vi "Transfer Multiple.vi"() -> ()   [LabVIEW 2020, in "Examples.lvlib"]
uses:
  Examples.lvlib
  Network Config/Network Config.lvclass
  Server Config/Server Config.lvclass
  PropertyBinder/Binding/Binding.lvclass/Binding.ctl
  PropertyBinder/Binding/Transfer.vi
  PropertyBinder/Binding/Set.vi
  PropertyBinder/Binding/Get.vi
  PropertyBinder/Binding/Binding.lvclass
panel:
  out "Time":dbl
  out "error out":errorcluster
  out "Bind Port":u16
  out "Bind Address":string
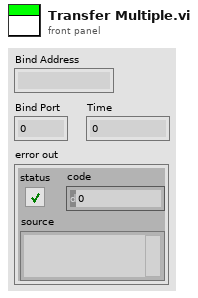
[diagram p1: front panel]
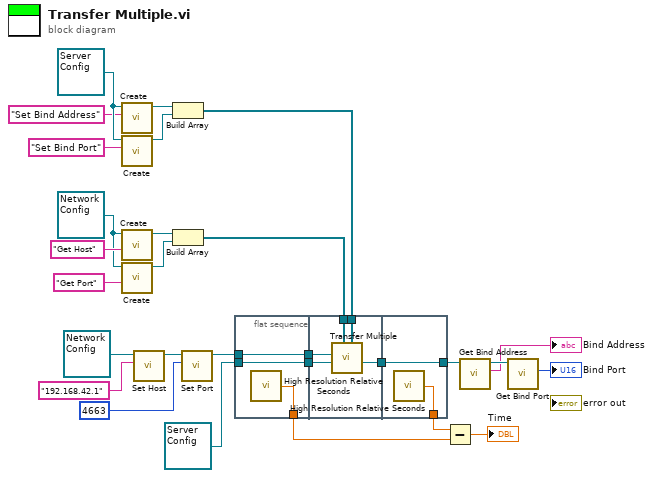
[diagram p0: block diagram]
diagram:
  w25 = refnum<class "Server Config.lvclass"> refnum ("Examples.lvlib:Server Config.lvclass")
  w26 = refnum<class "Network Config.lvclass"> refnum ("Examples.lvlib:Network Config.lvclass")
  n1 = call "Create.vi"("Setter VI Name"="Set Bind Address" ("Getter VI Name"), "Class Type"=w25) -> ("Binding out"=w11:refnum<class "Binding.lvclass">)  [unwired: 8 in, 1 out]
  n2 = call "Create.vi"("Setter VI Name"="Set Bind Port", "Class Type"=w25) -> ("Binding out"=w10:refnum<class "Binding.lvclass">)  [unwired: 8 in, 1 out]
  n3 = call "Create.vi"("Getter VI Name"="Get Host", "Class Type"=w26) -> ("Binding out"=w13:refnum<class "Binding.lvclass">)  [unwired: 8 in, 1 out]
  n4 = call "Create.vi"("Getter VI Name"="Get Port", "Class Type"=w26) -> ("Binding out"=w12:refnum<class "Binding.lvclass">)  [unwired: 8 in, 1 out]
  n5 = call "Set Host.vi"("Host"="192.168.42.1", "Network Config in"=refnum<class "Network Config.lvclass"> refnum ("Examples.lvlib:Network Config.lvclass")) -> ("Network Config out"=w20:refnum<class "Network Config.lvclass">)  [unwired: 8 in, 1 out]
  n6 = Build Array(w11, w10) -> (w8:refnum<class "Binding.lvclass">[])
  n7 = Build Array(w13, w12) -> (w9:refnum<class "Binding.lvclass">[])
  n8 = call "Set Port.vi"("Port"=u16 4663, "Network Config in"=w20) -> ("Network Config out"=w15:refnum<class "Network Config.lvclass">)  [unwired: 8 in, 1 out]
  n9 = flat-sequence {
    tunnel: refnum<class "Server Config.lvclass"> refnum ("Examples.lvlib:Server Config.lvclass") -> [w30]
    tunnel: w15 -> [w31]
    tunnel: [w31] -> w6
    tunnel: [w30] -> w5
    tunnel: [w29] -> w2
    tunnel: w9 -> [w34]
    tunnel: w8 -> [w33]
    tunnel: w6 -> [w36]
    tunnel: w5 -> [w35]
    tunnel: [w32] -> w4
    tunnel: [w38] -> w7
    tunnel: w4 -> [w38]
    tunnel: [w37] -> w3
    frame #0 {
      n10 = call <vilib>:"High Resolution Relative Seconds.vi"() -> ("relative seconds"=w29:dbl)
    }
    frame #1 {
      n11 = call "Transfer Multiple.vi"("To Bindings"=w33, "From Bindings"=w34, "To Class in"=w35, "From Class in"=w36) -> ("To Class out"=w32:refnum<class "Server Config.lvclass">)  [unwired: 5 in, 2 out]
    }
    frame #2 {
      n12 = call <vilib>:"High Resolution Relative Seconds.vi"() -> ("relative seconds"=w37:dbl)
    }
  }
  n13 = Subtract(x=w3, y=w2) -> (x-y=→"Time":dbl)
  n14 = call "Get Bind Address.vi"("Server Config in"=w7) -> ("Bind Address"=→"Bind Address":string, "Server Config out"=w18:refnum<class "Server Config.lvclass">)  [unwired: 8 in, 1 out]
  n15 = call "Get Bind Port.vi"("Server Config in"=w18) -> ("Bind Port"=→"Bind Port":u16)  [unwired: 8 in, 2 out]
